vi "send_trigger.vi"(8 "error in (no error)":errorcluster, 10 "message":T1, 11 "GenericScanMode in":refnum<class "GenericImagingMode.lvclass">) -> (0 "error out":errorcluster, 3 "GenericScanMode out":refnum<class "GenericImagingMode.lvclass">)   [LabVIEW 2010, in "GenericImagingMode.lvclass"]
uses:
  GenericImagingMode.lvclass
  trigger_enum.ctl
  common/classes/GenericToplevelComponent/GenericToplevelComponent/trigger_type_enum.ctl
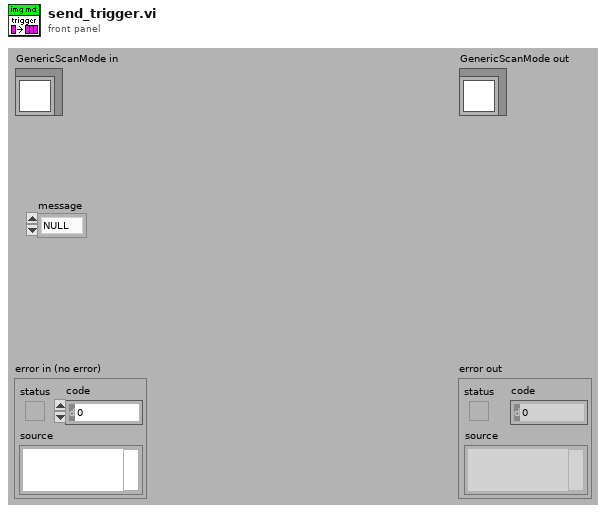
[diagram p1: front panel]
types:
  T1 = typedef "GenericImagingMode.lvclass/trigger_enum.ctl" = enum16{"NULL", "proceed"}
  T2 = typedef "trigger_type_enum.ctl" = enum8{"external", "internal", "common"}
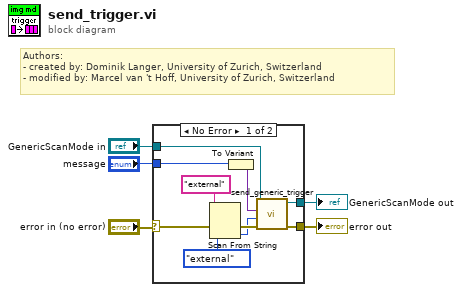
[diagram p0: block diagram]
diagram:
  # "Authors: \n- created by: Dominik Langer, University of Zurich, Switzerland\n- modified by: Marcel van 't Hoff, University of Zurich, Switzerland"
  n1 = case shown="No Error" "error in (no error)" {
    selector: "error in (no error)" -> [w9 w17]
    tunnel: [w12 w17] -> w5
    tunnel: [w13 w16] -> w1
    tunnel: "GenericScanMode in" -> [w14 w16]
    tunnel: "message" -> [w15 _]
    frame No Error {
      n2 = Scan From String(input string="external", error in=w9, default 1=trigger_type_enum."external" ("trigger type")) -> (error out=w8:errorcluster, output 1=w7:T2)  [unwired: 2 in, 2 out]
      n3 = To Variant(anything=w15) -> (Variant=w11:variant)
      n4 = call-dynamic "send_generic_trigger.vi"("error in (no error)"=w8, "trigger type"=w7, "trigger variant"=w11, "GenericToplevelComponent in"=w14) -> ("error out"=w12:errorcluster, "GenericToplevelComponent out"=w13:refnum<class "GenericImagingMode.lvclass">)  [unwired: 4 in, 2 out]
    }
    frame Error {
    }
  }
  "error out" <- w5
  "GenericScanMode out" <- w1
